vi "Destroy Reference.vi"(8 "Error In":errorcluster, 11 "Reader In":refnum<data-value>) -> (0 "Error Out":errorcluster, 3 "Reader Out":refnum<class "Reader.lvclass">)   [LabVIEW 2019, in "LabPack.lvlib" / "Reader.lvclass"]
doc: "Destroys a reference to a Reader class object. This may free resources associated with the reference but not necessarily the object."
uses:
  Reader.lvclass
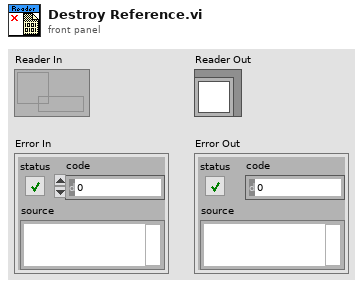
[diagram p1: front panel]
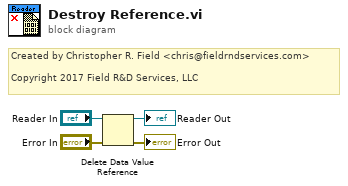
[diagram p0: block diagram]
diagram:
  # "Created by Christopher R. Field <chris@fieldrndservices.com>\n\nCopyright 2017 Field R&D Services, LLC"
  n1 = Delete Data Value Reference(data value reference="Reader In", error in="Error In") -> (data value=→"Reader Out":refnum<class "Reader.lvclass">, error out=→"Error Out":errorcluster)
